vi "Serial_puts.vi"(8 "error in (no error)":errorcluster, 9 "String":string, 11 "Serial.lvclass":refnum<class "Serial.lvclass">) -> (0 "error out":errorcluster, 3 "Serial.lvclass 2":refnum<class "Serial.lvclass">)   [LabVIEW 2011, in "mbed_LVLibrary.lvlib" / "Serial.lvclass"]
doc: "Writes the string to the serial port on mbed. Doesn't add a termination character so this should be included in the string"
uses:
  Serial.lvclass
  Serial.lvclass/Serial.ctl
  Transport Mechanisms/mbed/mbed.lvclass
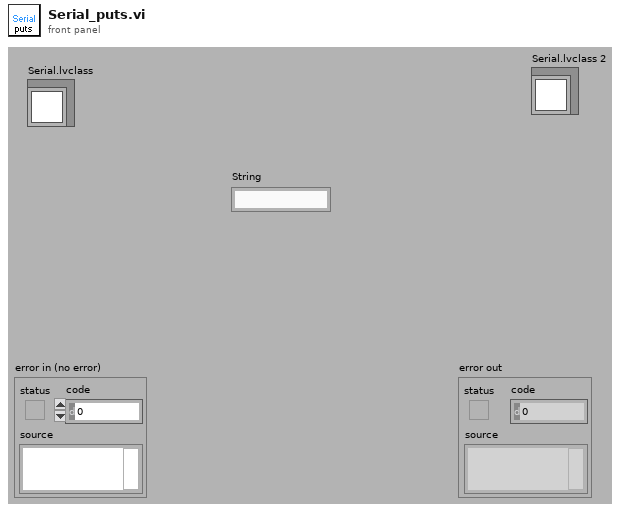
[diagram p1: front panel]
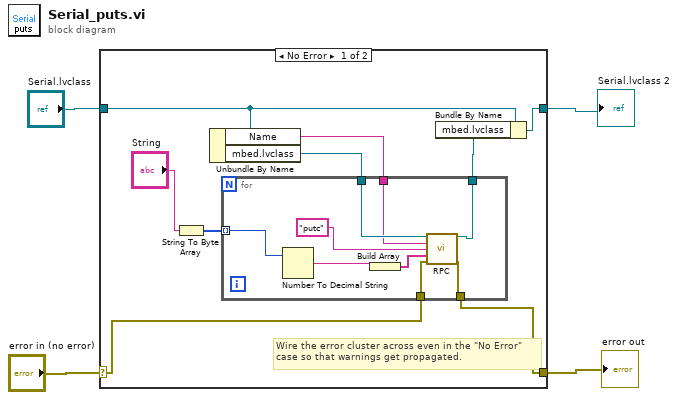
[diagram p0: block diagram]
diagram:
  n1 = case shown="No Error" "error in (no error)" {
    selector: "error in (no error)" -> [w6 w24]
    tunnel: [w5 w24] -> w3
    tunnel: [w8 w23] -> w1
    tunnel: "Serial.lvclass" -> [w9 w23]
    frame No Error {
      # "Wire the error cluster across even in the \"No Error\"\ncase so that warnings get propagated."
      n2 = String To Byte Array(string="String") -> (unsigned byte array=w10:u8[])
      n3 = Unbundle By Name(w9) -> ("Name"=w11:string, "mbed.lvclass"=w12:refnum<class "mbed.lvclass">)
      n4 = for {
        tunnel: w12 -> [w22]
        tunnel: w11 -> [w21]
        tunnel: w10 -> [w17] mode=indexing
        tunnel: [w16] -> w7
        tunnel: w6 -> [w15]
        tunnel: [w14] -> w5
        n5 = Number To Decimal String(number=w17) -> (decimal integer string=w18:string)  [unwired: 1 in]
        n6 = Build Array(w18) -> (w19:string[])
        n7 = call-dynamic "RPC.vi"("mbed in"=w22, "Name"=w21, "method"="putc", "Args"=w19, "error in (no error)"=w15) -> ("mbed out"=w16:refnum<class "mbed.lvclass">, "error out"=w14:errorcluster)  [unwired: 8 in, 1 out]
      }
      n8 = Bundle By Name(cluster=w9, "mbed.lvclass"=w7) -> (w8:refnum<class "Serial.lvclass">)
    }
    frame Error {
    }
  }
  "error out" <- w3
  "Serial.lvclass 2" <- w1
